vi "tidy up raw shot data array.vi"(11 "All shot data":string[][](array[string])=[["Cam1 shot #", "Cam1 exposure", "Cam1 trigger"], ["-1", "1.000000", "on"], ["Cam1 shot #", "Cam1 exposure", "Cam1 trigger"], ["-1", "1.000000", "on"], ["Cam1 shot #", "Cam1 exposure", "Cam1 trigger"], ["-1", "1.000000", "on"], ["Cam1 shot #", "Cam1 exposure", "Cam1 trigger"], ["-1", "1.000000", "on"], ["Cam1 shot #", "Cam1 exposure", "Cam1 trigger"], ["-1", "1.000000", "on"], ["Cam1 shot #", "Cam1 exposure", "Cam1 trigger"], ["-1", "1.000000", "on"], ["Cam1 shot #", "Cam1 exposure", "Cam1 trigger"], ["-1", "1.000000", "on"]]) -> (2 "Titles":string[](array[string]), 3 "output array":string[][](array[string]))   [LabVIEW 2009]
uses:
  <userlib>/_OpenG.lib/array/array.llb/Delete Elements from 2D Array (String)__ogtk.vi
  <userlib>/_OpenG.lib/array/array.llb/Search 1D Array (String)__ogtk.vi
panel:
  in  "scan data only":bool=TRUE
  out "data":string[][](array[string])
  out "Array":string[][](array[string])
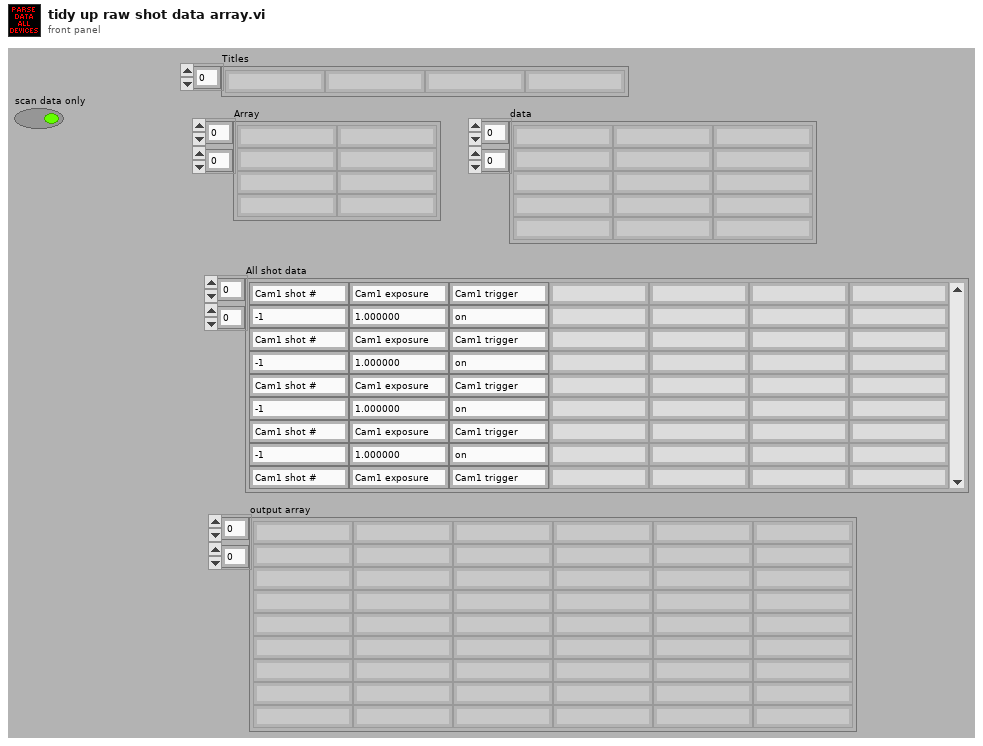
[diagram p1: front panel]
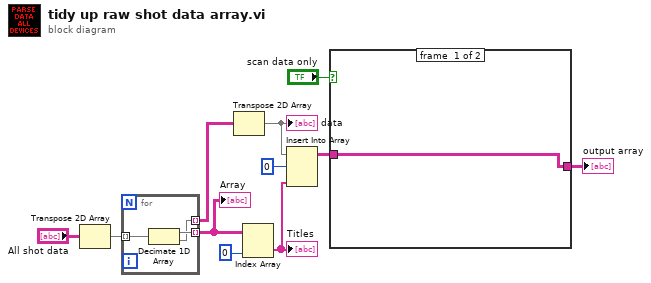
[diagram p0: block diagram]
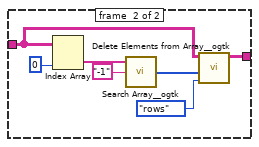
[diagram p2: hidden frame]
diagram:
  n1 = Transpose 2D Array(2D array="All shot data") -> (transposed array=w10:string[][])
  n2 = for {
    tunnel: w10 -> [w14] mode=indexing
    tunnel: [w13] -> w9 mode=indexing
    tunnel: [w12] -> w7 mode=indexing
    n3 = Decimate 1D Array(w14) -> (w13:string[], w12:string[])
  }
  "Array" <- w9
  n4 = Transpose 2D Array(2D array=w7) -> (transposed array=w4:string[][])
  "data" <- w4
  n5 = Index Array(array=w9, index (col)=0 ("disabled index (col)")) -> (element=w5:string[])  [unwired: 1 in]
  "Titles" <- w5
  n6 = Insert Into Array(array=w4, index (row)=0, new element=w5) -> (w3:string[][])  [unwired: 1 in]
  n7 = case shown="True" "scan data only" {
    tunnel: w3 -> [w15 w18]
    tunnel: [w15 w16] -> w2
    frame #0 {
    }
    frame #1 {
      n8 = Index Array(array=w18, index (col)=0 ("disabled index (col)")) -> (element=w21:string[])  [unwired: 1 in]
      n9 = call-poly <userlib>:"Search Array__ogtk.vi"("Array"=w21, "Element Data"="-1") -> ("Indices of Elements"=w19:i32[])  [unwired: 7 in]
      n10 = call-poly <userlib>:"Delete Elements from Array__ogtk.vi"("delete (rows or columns)"=enum16{"rows", "columns"}."rows", "indices"=w19, "array"=w18) -> ("array w/ subset deleted"=w16:string[][])  [unwired: 7 in, 1 out]
    }
  }
  "output array" <- w2
